vi "3.vi"() -> ()   [LabVIEW 2015]
uses:
  <vilib>/Utility/file.llb/Read Delimited Spreadsheet (string).vi
panel:
  out "User Level":string
  in  "User Name":string
  in  "User Level Cmd":T1(ring)
  out "Error Out":errorcluster
  in  "Error In":errorcluster
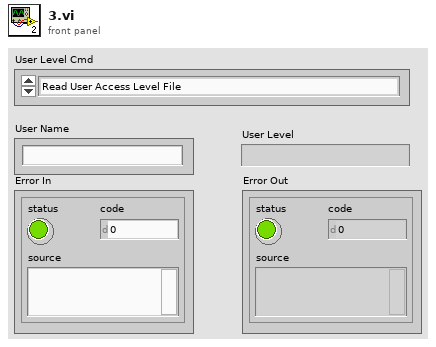
[diagram p1: front panel]
types:
  T1 = enum16{"Read User Access Level File", "Set Current User", "Get User Access Level"}
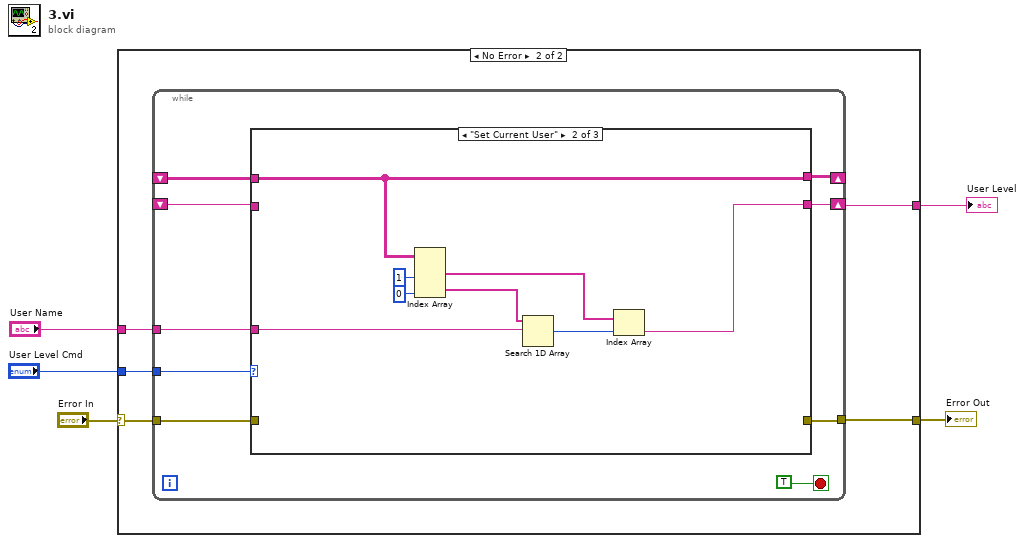
[diagram p0: block diagram]
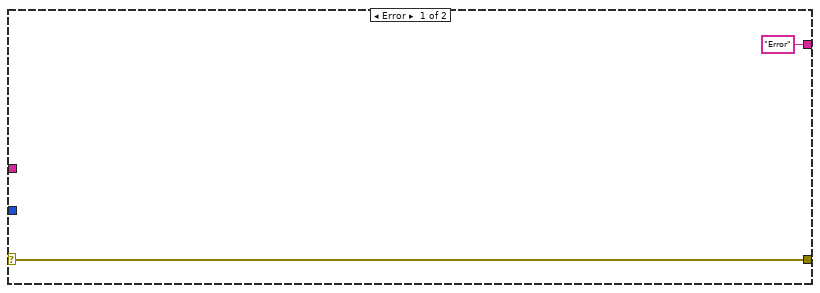
[diagram p2: hidden frame]
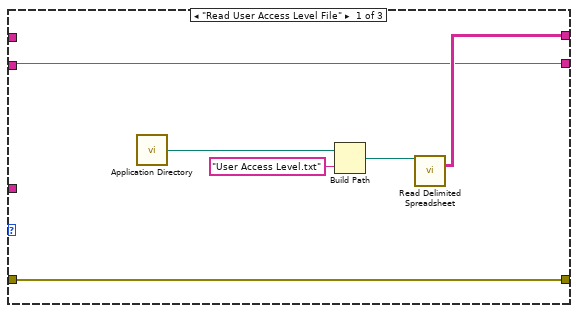
[diagram p3: hidden frame]
diagram:
  n1 = case shown="No Error" "Error In" {
    selector: "Error In" -> [w7 w12]
    tunnel: [w7 w11] -> w4
    tunnel: "User Name" -> [_ w10]
    tunnel: "User Level Cmd" -> [_ w9]
    tunnel: ["Error" ("String") w8] -> w1
    frame Error {
    }
    frame No Error {
      n2 = while {
        tunnel: w12 -> [w21]
        tunnel: [w20] -> w11
        tunnel: w10 -> [w18]
        tunnel: w9 -> [w17]
        shift-right: [w16] -> _
        shift-left: _ -> [w15]
        shift-right: [w14] -> w8
        shift-left: _ -> [w13]
        stop <- TRUE stop-if-true
        n3 = case shown="\"Set Current User\"" w17 {
          tunnel: w21 -> [w27 _ _]
          tunnel: [w27 _ _] -> w20
          tunnel: w18 -> [_ w32 _]
          tunnel: [w23 w33 w36] -> w16
          tunnel: w15 -> [_ w33 w36]
          tunnel: w13 -> [w22 _ _]
          tunnel: [w22 w34 _] -> w14
          frame "Read User Access Level File" {
            n4 = call <vilib>:"Application Directory.vi"() -> ("Application Directory"=w25:path)
            n5 = Build Path(base path=w25, name or relative path="User Access Level.txt") -> (appended path=w24:path)
            n6 = call-poly <vilib>:"Read Delimited Spreadsheet.vi"("file path (dialog if empty)"=w24) -> ("all rows"=w23:string[][])  [unwired: 9 in, 5 out]
          }
          frame "Set Current User" {
            n7 = Index Array "Index Array"(array=w33, index (col) #1=1 ("disabled index (col)"), index (col) #2=0 ("index (col)")) -> (element #1=w30:string[], element #2=w31:string[])  [unwired: 2 in]
            n8 = Search 1D Array(1D array=w31, element=w32) -> (index of element=w35:i32)  [unwired: 1 in]
            n9 = Index Array "Index Array"(array=w30, index=w35) -> (element=w34:string)
          }
          frame "Get User Access Level" {
          }
        }
      }
    }
  }
  "Error Out" <- w4
  "User Level" <- w1
